vi "Input_Generator.vi"(9 "Input Offsets":dbl[](array[numeric]), 10 "Input Gains":dbl[](array[numeric]), 11 "Input Vector":dbl[](array[numeric])) -> (3 "To Mossy Fibers":dbl[](array[numeric]))   [LabVIEW 2016]
panel:
  out "Inputs to Mossy Fibers":T1(graph)
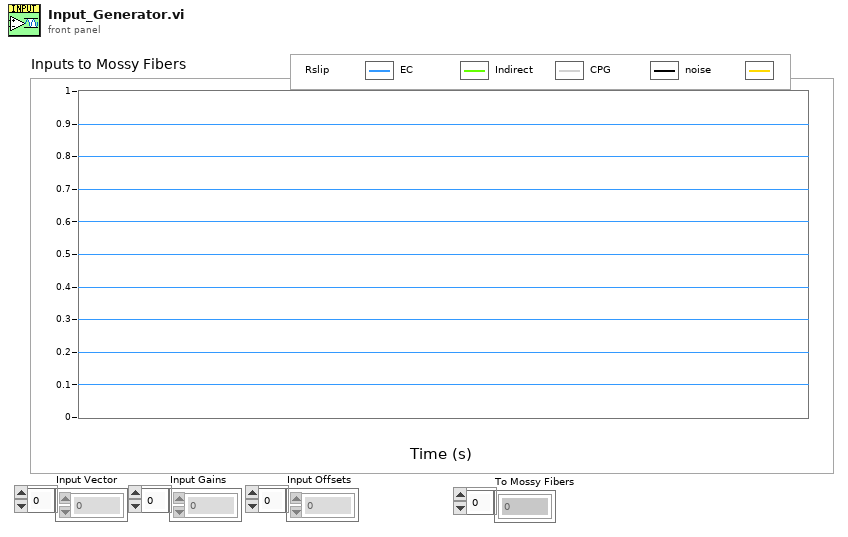
[diagram p1: front panel]
types:
  T1 = cluster{"[0]":dbl, "[1]":dbl, "[2]":dbl, "[3]":dbl, "[4]":dbl, "[5]":dbl, "[6]":dbl, "[7]":dbl, "[8]":dbl}
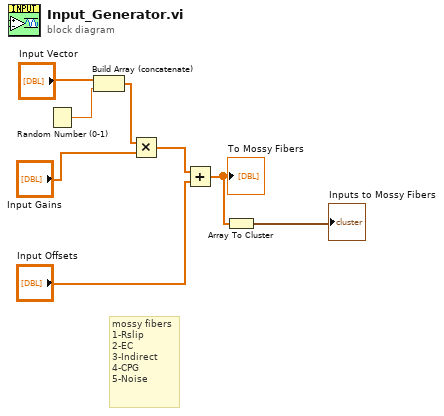
[diagram p0: block diagram]
diagram:
  # "mossy fibers\n1-Rslip\n2-EC\n3-Indirect\n4-CPG\n5-Noise"
  n1 = Random Number (0-1)() -> (number: 0 to 1=w7:dbl)
  n2 = Build Array (concatenate)("Input Vector", w7) -> (w2:dbl[])
  n3 = Multiply(x=w2, y="Input Gains") -> (x*y=w1:dbl[])
  n4 = Add(x=w1, y="Input Offsets") -> (x+y=w4:dbl[])
  "To Mossy Fibers" <- w4
  n5 = Array To Cluster(array=w4) -> (cluster=→"Inputs to Mossy Fibers":T1)
